vi "LF2R IDE Cmd.vi"(8 "error in (no error)":errorcluster, 9 "Data":variant, 10 "CMD":T1, 11 "LF2R IDE in":refnum<class "LF2R IDE.lvclass">) -> (0 "error out":errorcluster, 3 "LF2R IDE out":refnum<class "LF2R IDE.lvclass">)   [LabVIEW 2018, in "LF2R IDE.lvlib" / "LF2R IDE.lvclass"]
uses:
  LF2R IDE.lvclass
  LF2R IDE Cmd.ctl
  LF2R IDE Cmd Data.ctl
  LF2R IDE.lvclass/LF2R IDE.ctl
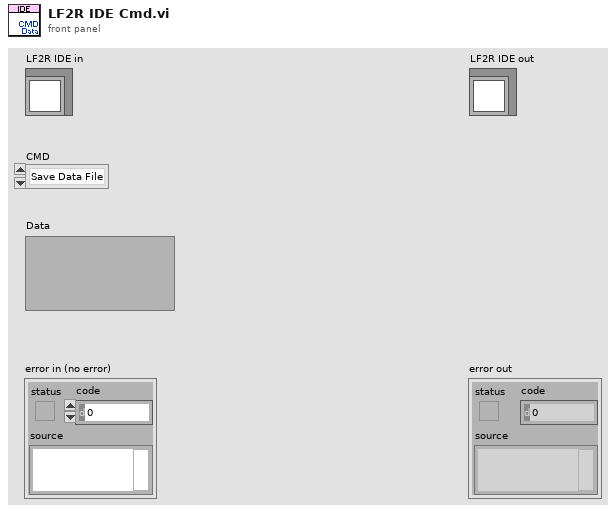
[diagram p1: front panel]
types:
  T1 = typedef "LF2R IDE.lvlib/LF2R IDE.lvclass/LF2R IDE Cmd.ctl" = enum16{"Save Data File", "Write Configuration", "Update Frame Image"}
  T2 = typedef "LF2R IDE.lvlib/LF2R IDE.lvclass/LF2R IDE Cmd Data.ctl" = cluster{"CMD":T1, "Data":variant}
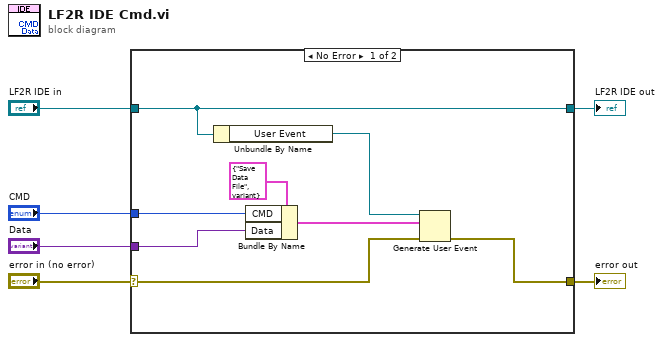
[diagram p0: block diagram]
diagram:
  n1 = case shown="No Error" "error in (no error)" {
    selector: "error in (no error)" -> [w8 w16]
    tunnel: [w7 w16] -> w5
    tunnel: [w11 w15] -> w3
    tunnel: "LF2R IDE in" -> [w11 w15]
    tunnel: "CMD" -> [w13 _]
    tunnel: "Data" -> [w12 _]
    frame No Error {
      n2 = Unbundle By Name(w11) -> ("User Event"=w10:refnum<user-event>)
      n3 = Bundle By Name(cluster=T2 {"CMD"=enum."Save Data File", "Data"=variant} ("CMDData"), "CMD"=w13, "Data"=w12) -> (w9:T2)
      n4 = Generate User Event(user event=w10, event data cluster=w9, error in=w8) -> (error out=w7:errorcluster)  [unwired: 1 in, 1 out]
    }
    frame Error {
    }
  }
  "error out" <- w5
  "LF2R IDE out" <- w3
